vi "SLSC Coerce Number to ENUM.vi"(7 "Default Enum":i32, 9 "enums":T1[](array[typedef]), 10 "Enum in":i32, 11 "dataType":string) -> (2 "Found?":bool, 3 "Enum out":i32)   [LabVIEW 2017, in "SLSC EDS System Explorer.lvlib"]
uses:
  SLSC EDS System Explorer.lvlib
  SLSC EDS API/JSON parsing/enum.ctl
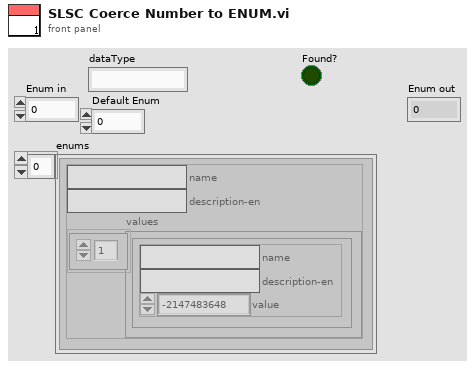
[diagram p1: front panel]
types:
  T1 = typedef "enum.ctl" = cluster{"name":string, "description-en":string, "values":cluster{"name":string, "description-en":string, "value":i32}[]}
  T2 = cluster{"name":string, "description-en":string, "value":i32}[]
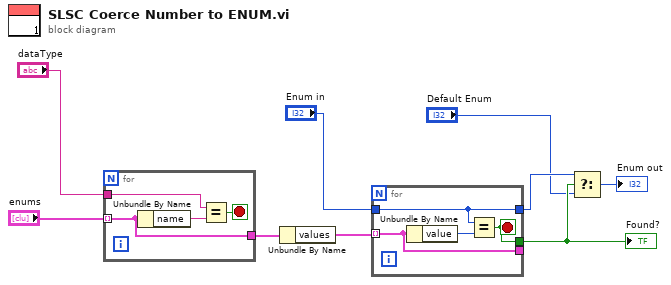
[diagram p0: block diagram]
diagram:
  n1 = for {
    tunnel: "enums" -> [w11] mode=indexing
    tunnel: "dataType" -> [w12]
    tunnel: [w11] -> w7
    stop <- w10 stop-if-true
    n2 = Unbundle By Name(w11) -> ("name"=w13:string)
    n3 = Equal?(x=w12, y=w13) -> (x = y?=w10:bool)
  }
  n4 = Unbundle By Name(w7) -> ("values"=w6:T2)
  n5 = for {
    tunnel: w6 -> [w16] mode=indexing
    tunnel: "Enum in" -> [w15]
    tunnel: [w16] -> _
    tunnel: [w15] -> w3
    tunnel: [w14] -> w4
    stop <- w14 stop-if-true
    n6 = Unbundle By Name(w16) -> ("value"=w17:i32)
    n7 = Equal?(x=w15, y=w17) -> (x = y?=w14:bool)
  }
  "Found?" <- w4
  n8 = Select(t=w3, s=w4, f="Default Enum") -> (s? t:f=→"Enum out":i32)
